vi "camera globals.vi"() -> ()   [LabVIEW 2016]
uses:
  ixon camera/HAL camera properties.ctl
panel:
  in  "Camera Properties":T1
  in  "Number of acquisition blocks":i8(slide)=10 scale=0.0..20.0
  in  "Camera Acquiring":bool
  # "Camera:  Andor iXon/iXon Ultra"
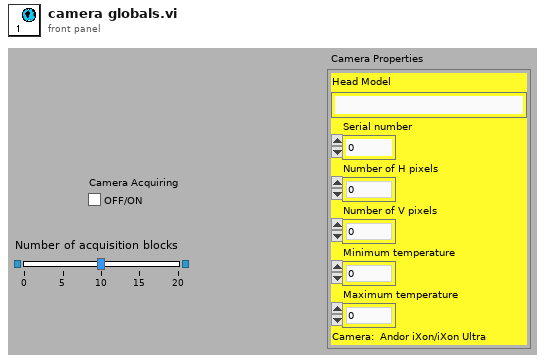
[diagram p1: front panel]
types:
  T1 = typedef "HAL camera properties.ctl" = cluster{"Head Model":string, "Serial number":i32, "Number of H pixels":i32, "Number of V pixels":i32, "Minimum temperature":i32, "Maximum temperature":i32}
diagram:
